vi "send_trigger.vi"(8 "error in (no error)":errorcluster, 10 "trigger":T1, 11 "GenericImageAssembler in":refnum<class "GenericImageAssembler.lvclass">) -> (0 "error out":errorcluster, 3 "GenericImageAssembler out":refnum<class "GenericImageAssembler.lvclass">)   [LabVIEW 2010, in "GenericImageAssembler.lvclass"]
uses:
  GenericImageAssembler.lvclass
  trigger_enum.ctl
  common/classes/GenericToplevelComponent/GenericToplevelComponent/trigger_type_enum.ctl
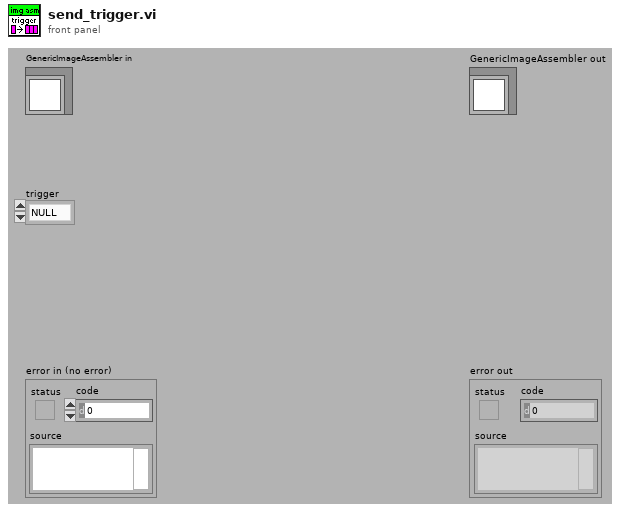
[diagram p1: front panel]
types:
  T1 = typedef "GenericImageAssembler.lvclass/trigger_enum.ctl" = enum16{"NULL", "start", "stop"}
  T2 = typedef "trigger_type_enum.ctl" = enum8{"external", "internal", "common"}
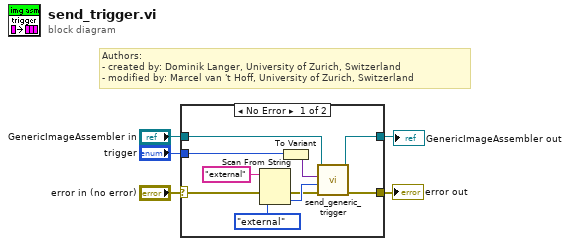
[diagram p0: block diagram]
diagram:
  # "Authors: \n- created by: Dominik Langer, University of Zurich, Switzerland\n- modified by: Marcel van 't Hoff, University of Zurich, Switzerland"
  n1 = case shown="No Error" "error in (no error)" {
    selector: "error in (no error)" -> [w8 w16]
    tunnel: [w14 w17] -> w4
    tunnel: "GenericImageAssembler in" -> [w13 w17]
    tunnel: "trigger" -> [w12 _]
    tunnel: [w15 w16] -> w5
    frame No Error {
      n2 = Scan From String(input string="external", error in=w8, default 1=trigger_type_enum."external" ("trigger type")) -> (error out=w7:errorcluster, output 1=w9:T2)  [unwired: 2 in, 2 out]
      n3 = To Variant(anything=w12) -> (Variant=w11:variant)
      n4 = call-dynamic "send_generic_trigger.vi"("error in (no error)"=w7, "trigger type"=w9, "trigger variant"=w11, "GenericToplevelComponent in"=w13) -> ("error out"=w15:errorcluster, "GenericToplevelComponent out"=w14:refnum<class "GenericImageAssembler.lvclass">)  [unwired: 4 in, 2 out]
    }
    frame Error {
    }
  }
  "error out" <- w5
  "GenericImageAssembler out" <- w4
